vi "Multi-line String to Array.vi"(1 "Multi lined string":string) -> (0 "Array of string lines":string[](array[string]))   [LabVIEW 2011]
doc: "Converts a multiline input <B>string</B> to a 1D array of <B>lines</B> (without EOLs). If the input string ends in an EOL, then the last line will be removed (since it is empty) -- this behavior is useful for instrument communication where the last line ends with a EOL character that we do not wish to treat as a seperate line (since it contains no data)."
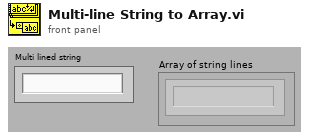
[diagram p1: front panel]
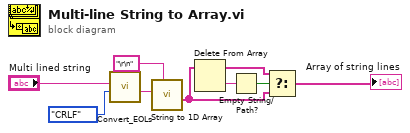
[diagram p0: block diagram]
diagram:
  n1 = call "Convert_EOLs.vi"("Convert to:"=enum16{"CR", "LF", "CRLF"}."CRLF", "String in"="Multi lined string") -> ("String out"=w3:string)  [unwired: 9 in]
  n2 = call "String to 1D Array.vi"("delimiter (Tab)"="\r\n", "string"=w3) -> ("Array of Strings"=w8:string[])  [unwired: 9 in]
  n3 = Delete From Array(array=w8) -> (deleted portion=w7:string, array with subset deleted=w6:string[])  [unwired: 2 in]
  n4 = Empty String/Path?(string/path=w7) -> (empty?=w5:bool)
  n5 = Select(t=w6, s=w5, f=w8) -> (s? t:f=→"Array of string lines":string[])
